vi "Rx String Concatenate.vi"(0 "Input Rx Message":string, 5 "error in":errorcluster) -> (4 "Output Rx Message":string, 6 "error out":errorcluster)   [LabVIEW 2012, in "UART_Host_Driver.lvlib" / "UART Driver.lvclass"]
uses:
  UART Driver.lvclass
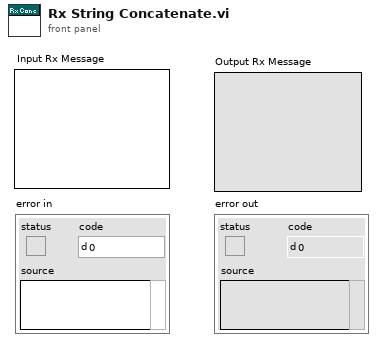
[diagram p1: front panel]
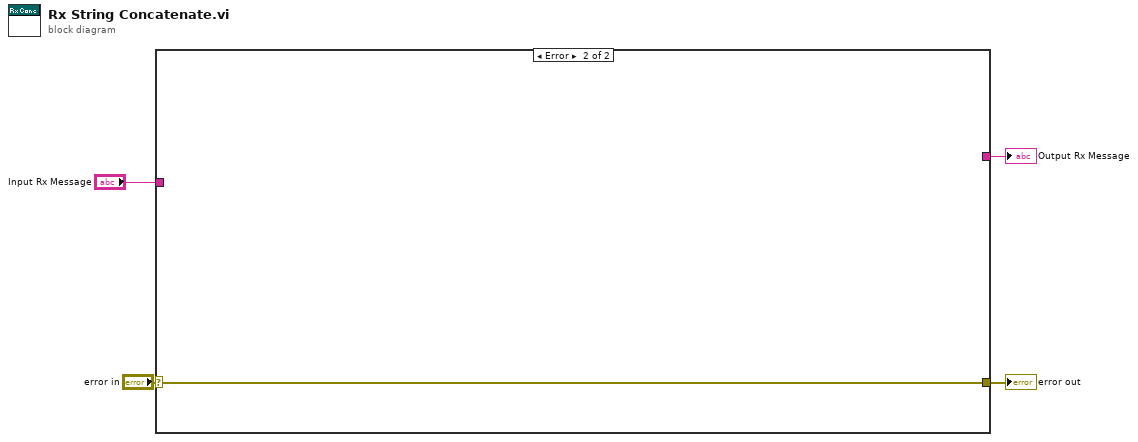
[diagram p0: block diagram]
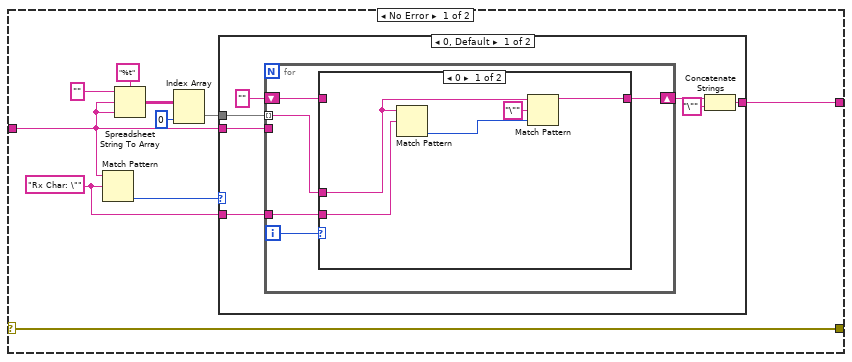
[diagram p2: hidden frame]
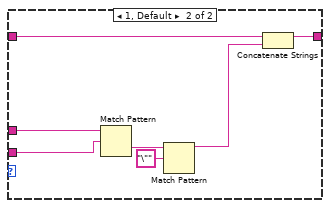
[diagram p3: hidden frame]
diagram:
  n1 = case shown="Error" "error in" {
    selector: "error in" -> [w14 w40]
    tunnel: [w14 w40] -> w3
    tunnel: "Input Rx Message" -> [w8 _]
    tunnel: [w5 _] -> w1
    frame No Error {
      w7 = "Rx Char: \"" ("regular expression")
      n2 = Match Pattern(string=w8, regular expression=w7) -> (offset past match=w6:i32)  [unwired: 1 in, 3 out]
      n3 = Spreadsheet String To Array(delimiter (Tab)="%t", format string="", spreadsheet string=w8, array type (2D Dbl)=w8) -> (array=w11:string[][])
      n4 = Index Array(array=w11, index (col)=0 ("disabled index (col)")) -> (element=w9:string[])  [unwired: 1 in]
      n5 = case shown="0, Default" w6 {
        tunnel: w8 -> [w21 w39]
        tunnel: [w16 w39] -> w5
        tunnel: w9 -> [w18 _]
        tunnel: w7 -> [w17 _]
        frame 0, Default {
          n6 = for {
            tunnel: w21 -> [_]
            shift-right: [w25] -> w19
            shift-left: "" -> [w24]
            tunnel: w18 -> [w23] mode=indexing
            tunnel: w17 -> [w22]
            i -> [w26]
            n7 = case shown="0" w26 {
              tunnel: [w27 w35] -> w25
              tunnel: w24 -> [_ w37]
              tunnel: w23 -> [w28 w34]
              tunnel: w22 -> [w30 w33]
              frame 0 {
                n8 = Match Pattern(string=w28, regular expression=w30) -> (offset past match=w29:i32)  [unwired: 1 in, 3 out]
                n9 = Match Pattern(string=w28, regular expression="\"", offset (0)=w29) -> (before substring=w27:string)  [unwired: 3 out]
              }
              frame 1, Default {
                n10 = Match Pattern(string=w34, regular expression=w33) -> (after substring=w32:string)  [unwired: 1 in, 3 out]
                n11 = Match Pattern(string=w32, regular expression="\"") -> (before substring=w36:string)  [unwired: 1 in, 3 out]
                n12 = Concatenate Strings(w37, w36) -> (w35:string)
              }
            }
          }
          n13 = Concatenate Strings(w19, "\"" ("string")) -> (w16:string)
        }
        frame -1 {
        }
      }
    }
    frame Error {
    }
  }
  "Output Rx Message" <- w1
  "error out" <- w3
